vi "4_颜色识别.vi"() -> ()   [LabVIEW 2020]
uses:
  <vilib>/vision/NI_Vision_Development_Module.lvlib
panel:
  out "黄色":bool
  out "红色":bool
  out "绿色":bool
  in  "停止":bool
  out "Color Spectrum":dbl[](array[numeric]) format="%.2f"
  out "error out":errorcluster
  in  "Rectangle":T1 {"Rotation" min=-90.0 max=90.0 step=1.0 format="%.2f"; "Left" scale=0.0..1024.0; "Right" scale=0.0..1024.0}
  out "Image":T2(plugin-control)
  in  "File Path":path
  in  "Image Type":T3 items=["Grayscale (U8)", "Grayscale (I16)", "Grayscale (SGL)", "Complex (CSG)", "RGB (U32)", "HSL (U32)", "RGB (U64)", "Grayscale (U16)"]
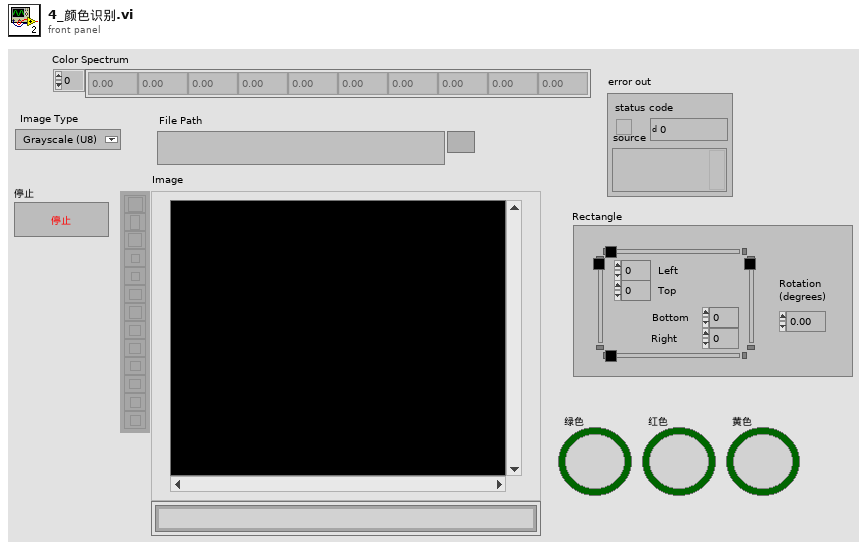
[diagram p1: front panel]
types:
  T1 = typedef "IMAQ Rectangle" = cluster{"Left":i32, "Top":i32, "Right":i32, "Bottom":i32, "Rotation":dbl}
  T2 = typedef "IMAQ Image.ctl" = refnum<image>
  T3 = typedef "Image Type" = u32
  T4 = typedef "ROI Descriptor" = cluster{"Global Rectangle":i32[], "Contours":cluster{"ID":enum32{"External", "Internal"}, "Type":u32, "Coordinates":i32[]}[]}
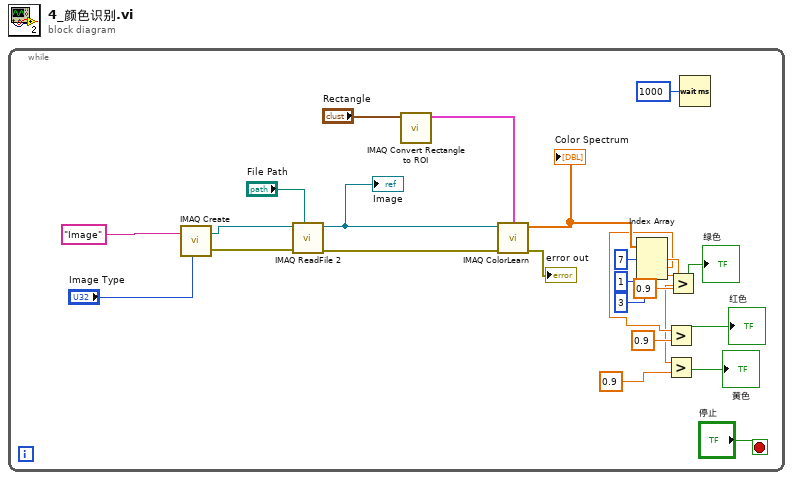
[diagram p0: block diagram]
diagram:
  n1 = while {
    stop <- "停止" stop-if-true
    n2 = call "IMAQ Create"("Image Name"="Image", "Image Type"="Image Type") -> ("New Image"=w21:T2, "error out"=w23:errorcluster)  [unwired: 3 in]
    n3 = call "IMAQ ReadFile 2"("File Path"="File Path", "error in (no error)"=w23, "Image"=w21) -> ("error out"=w22:errorcluster, "Image Out"=w19:T2)  [unwired: 4 in, 3 out]
    "Image" <- w19
    n4 = call "IMAQ Convert Rectangle to ROI"("Rectangle"="Rectangle") -> ("ROI Descriptor"=w18:T4)  [unwired: 8 in, 1 out]
    n5 = call "IMAQ ColorLearn"("ROI Descriptor"=w18, "Image"=w19, "error in (no error)"=w22) -> ("Color Spectrum"=w12:dbl[], "error out"=→"error out":errorcluster)  [unwired: 5 in]
    "Color Spectrum" <- w12
    n6 = Index Array(array=w12, index #1=7 ("索引"), index #2=1 ("索引"), index #3=3 ("索引")) -> (element #1=w11:dbl, element #2=w2:dbl, element #3=w1:dbl)
    n7 = Greater?(x=w2, y=0.9) -> (0:→"红色":bool)
    n8 = Greater?(x=w1, y=0.9) -> (0:→"黄色":bool)
    n9 = Greater?(x=w11, y=0.9) -> (0:→"绿色":bool)
    n10 = Wait (ms)(milliseconds to wait=u32 1000 ("等待时间（毫秒）")) -> ()  [unwired: 1 out]
  }
